vi "checkCallback.vi"(8 "error in (no error)":errorcluster, 11 "SALCommunicator in":refnum<class "SALCommunicatorDL.lvclass">) -> (0 "error out":errorcluster, 3 "SALCommunicator out":refnum<class "SALCommunicatorDL.lvclass">)   [LabVIEW 2016, in "SALCommunicatorDL.lvclass"]
uses:
  SALCommunicatorDL.lvclass
  ts_sallv_exa/SALLV_EXA.lvlib
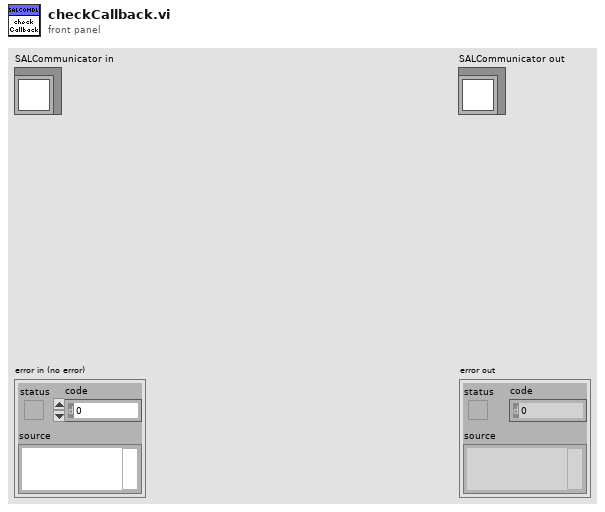
[diagram p1: front panel]
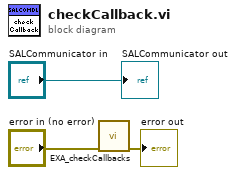
[diagram p0: block diagram]
diagram:
  n1 = call "EXA_checkCallbacks.vi"("error in (no error)"="error in (no error)") -> ("error out"=→"error out":errorcluster)  [unwired: 10 in]
  "SALCommunicator out" <- "SALCommunicator in"
